vi "SSC Relay Control Single Action.vi"(0 "SSC Relay in":T1[](array[typedef]), 5 "Relay Action":T3=21 items=["Open Relay"=20, "Close Relay"=21], 7 "Settling Time (s)":dbl, 11 "error in":errorcluster) -> (4 "SSC Relay out":T1[](array[typedef]), 8 "Completed Relay Operations":T2[](array[typedef]) {"Desired State" items=["Open Relay"=20, "Close Relay"=21]}, 15 "error out":errorcluster)   [LabVIEW 2019]
doc: "Performs the specified relay action on all Relays configured in the SSC Relay session. The function will then wait a specified amount of time if the Settling Time (s) input is wired."
uses:
  <instrlib>/niSwitch/niSwitch.llb/niSwitch Relay Action.ctl
  SSC Relay.ctl
  SubVIs/TSM Relay Completed Operations.ctl
  Single SSC Relay NI-Switch Control.vi
  Single SSC Relay Fill Additional Error info.vi
  SSC Relay Expand Action Array to All Sessions.vi
  <vilib>/Utility/error.llb/Error Cluster From Error Code.vi
  <instrlib>/niSwitch/niSwitch.llb/niSwitch Get Relay Position.vi
  <instrlib>/niSwitch/niSwitch.llb/niSwitch Relay Control.vi
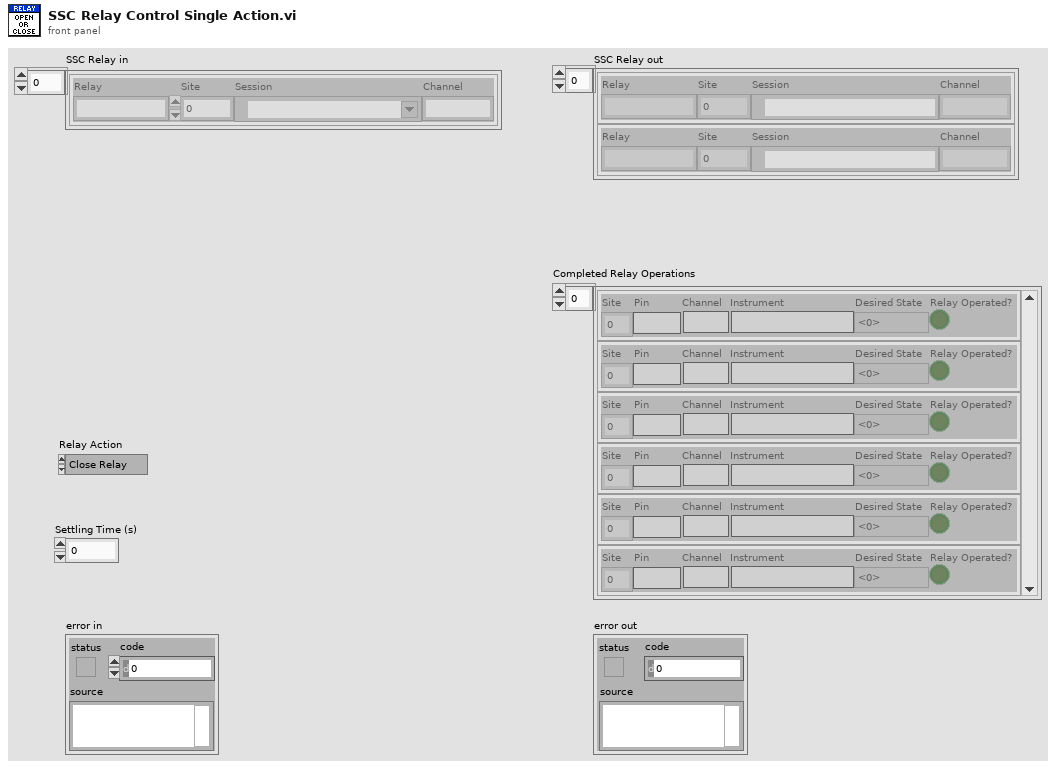
[diagram p1: front panel]
types:
  T1 = typedef "SSC Relay.ctl" = cluster{"Relay":string, "Site":i32, "Session":refnum<k15>, "Channel":string}
  T2 = typedef "TSM Relay Completed Operations.ctl" = cluster{"Site":i32, "Pin":string, "Channel":string, "Instrument":string, "Desired State":T3, "Relay Operated?":bool}
  T3 = typedef "niSwitch Relay Action.ctl" = i32
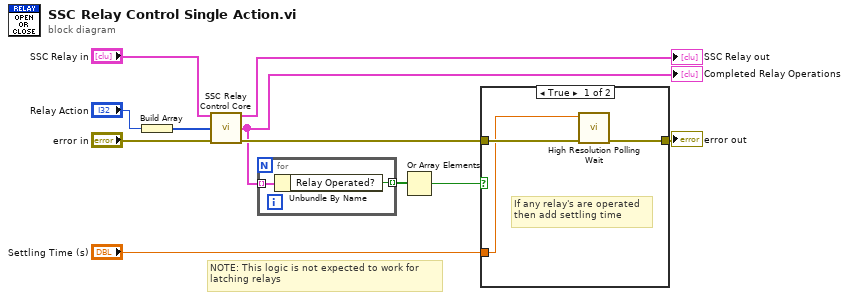
[diagram p0: block diagram]
diagram:
  # "NOTE: This logic is not expected to work for\nlatching relays"
  n1 = Build Array("Relay Action") -> (w7:T3[])
  n2 = call "SSC Relay Control Core.vi"("SSC Relay in"="SSC Relay in", "Relay Commands"=w7, "error in"="error in") -> ("SSC Relay out"=→"SSC Relay out":T1[], "Completed Relay Operations"=w3:T2[], "error out"=w9:errorcluster)  [unwired: 10 in]
  "Completed Relay Operations" <- w3
  n3 = for {
    tunnel: w3 -> [w13] mode=indexing
    tunnel: [w12] -> w2 mode=indexing
    n4 = Unbundle By Name(w13) -> ("Relay Operated?"=w12:bool)
  }
  n5 = Or Array Elements(Boolean array=w2) -> (logical OR=w1:bool)
  n6 = case shown="True" w1 {
    tunnel: [w16 w17] -> w11
    tunnel: w9 -> [w15 w17]
    tunnel: "Settling Time (s)" -> [w14 _]
    frame True {
      # "If any relay's are operated \nthen add settling time"
      n7 = call <vilib>:"High Resolution Polling Wait.vi"("error in (no error)"=w15, "seconds to wait"=w14) -> ("error out"=w16:errorcluster)  [unwired: 9 in]
    }
    frame False {
      # "If relays are not operated"
    }
  }
  "error out" <- w11
